vi "CalculateCS_TerminalHalfHeight.vi"(8 "error in (no error)":errorcluster, 11 "OuterTerminal":refnum<vi>) -> (0 "error out":errorcluster, 2 "CS outer terminal half-height":i32, 3 "OuterTerminal (dup)":refnum<vi>)   [LabVIEW 2017, in "ErrorStructureDrawer.lvlib"]
doc: "Calculates half of the height of the specified case structure outer terminal"
uses:
  ErrorStructureDrawer.lvlib
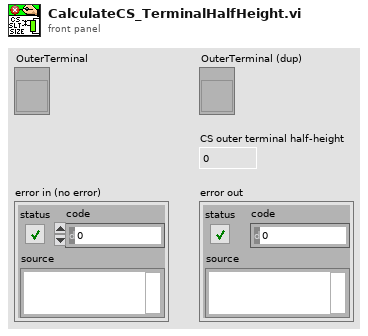
[diagram p1: front panel]
types:
  T1 = typedef "LVRectTypeDef.ctl" = cluster{"Left":i16, "Top":i16, "Right":i16, "Bottom":i16}
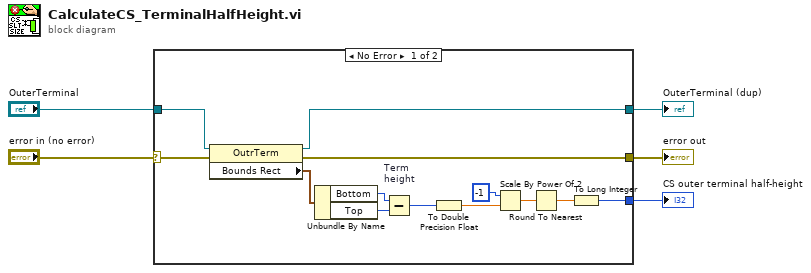
[diagram p0: block diagram]
diagram:
  n1 = case shown="No Error" "error in (no error)" {
    selector: "error in (no error)" -> [w6 w20]
    tunnel: [w18 w19] -> w5
    tunnel: [w17 w20] -> w4
    tunnel: "OuterTerminal" -> [w16 w19]
    tunnel: [w15 _] -> w2
    frame No Error {
      n2 = property class="OutrTerm"(reference=w16, error in=w6) -> (reference out=w18:refnum<vi>, error out=w17:errorcluster, "Bounds Rect"=w14:T1)
      n3 = Unbundle By Name(w14) -> ("Bottom"=w7:i16, "Top"=w13:i16)
      n4 = Subtract "Term \nheight"(x=w7, y=w13) -> (x-y=w8:i16)
      n5 = To Double Precision Float(number=w8) -> (double precision float=w9:dbl)
      n6 = Scale By Power Of 2(n=i16 -1, x=w9) -> (x*2^n=w11:dbl)
      n7 = Round To Nearest(number=w11) -> (nearest integer value=w12:dbl)
      n8 = To Long Integer(number=w12) -> (32bit integer=w15:i32)
    }
    frame Error {
    }
  }
  "OuterTerminal (dup)" <- w5
  "error out" <- w4
  "CS outer terminal half-height" <- w2
